vi "Format VI Info Table.vi"(5 "Type":T1=enum."LLB", 7 "Methods":T2, 8 "Error in":errorcluster caption="Error in (no error)", 9 "Msg Chain":string, 10 "VI Info Array":T3[](array[typedef]), 11 "VIDoc Printer - Confluence In":refnum<class "VIDoc Printer - Confluence.lvclass">) -> (0 "Error out":errorcluster, 2 "Table String":string, 3 "VIDoc Printer - Confluence Out":refnum<class "VIDoc Printer - Confluence.lvclass">)   [LabVIEW 2023, in "VIDoc Printer - Confluence.lvlib" / "VIDoc Printer - Confluence.lvclass"]
uses:
  VIDoc Printer - Confluence.lvclass
  Parsing/TypeDefs/Method Spec Cluster.ctl
  Parsing/TypeDefs/VI Type Extended Enum.ctl
  <vilib>/picture/picture.llb/imagedata.ctl
  Parsing/TypeDefs/Class Dispatch Type Enum.ctl
  Parsing/TypeDefs/Controls Info Cluster.ctl
  <vilib>/Utility/miscctls.llb/LVKeyTypeDef.ctl
  <vilib>/Utility/miscctls.llb/LVPointTypeDef.ctl
  Parsing/SubVIs/Structure Reporter/Tree Cluster.ctl
  Settings/Printer Settings/Detail Level Enum.ctl
  C:/projects/DMC/GitHub/DMC CLI VIDoc/Source/Documentation Generation/Printers/Printer/VIDoc Printer.lvclass
  Types/VI Method Types.ctl
  Printer/VIDoc Printer.lvclass/VIDoc Printer.ctl
  VIDoc Printer - Confluence.lvclass/VIDoc Printer - Confluence.ctl
  Types/VI Info Image Types.ctl
  Accessors/Get Method List Column Ordering - Minimal.vi
  Accessors/Get UI Column Ordering - Minimal.vi
  Accessors/Get VI Method Column Ordering - Minimal.vi
  Accessors/Get Class Method Column Ordering - Minimal.vi
  Accessors/Get Library Method Column Ordering - Minimal.vi
  Accessors/Get Interface Column Ordering - Minimal.vi
  Accessors/Get Method List Column Ordering - Standard.vi
  Accessors/Get UI Column Ordering - Standard.vi
  Accessors/Get VI Method Column Ordering - Standard.vi
  Accessors/Get Class Method Column Ordering - Standard.vi
  Accessors/Get Library Method Column Ordering - Standard.vi
  Accessors/Get Interface Column Ordering - Standard.vi
  Accessors/Get Method List Column Ordering - Full.vi
  Accessors/Get Library Method Column Ordering - Full.vi
  Accessors/Get UI Column Ordering - Full.vi
  Accessors/Get VI Method Column Ordering - Full.vi
  Accessors/Get Interface Column Ordering - Full.vi
  Accessors/Get Class Method Column Ordering - Full.vi
  Printer/Accessors/Get Formatting Settings.vi
  Accessors/Get Sortable Tables.vi
  Printer/VIDoc Printer.lvclass
  Confluence Formatting/Confluence Formatting.lvlib
  UI Interaction/UI Interaction.lvclass
  Parsing/VIDoc Parsing.lvlib
  Settings/Printer Settings/Printer Settings.lvclass
  Parsing/SubVIs/Structure Reporter/Structure Reporter.lvlib
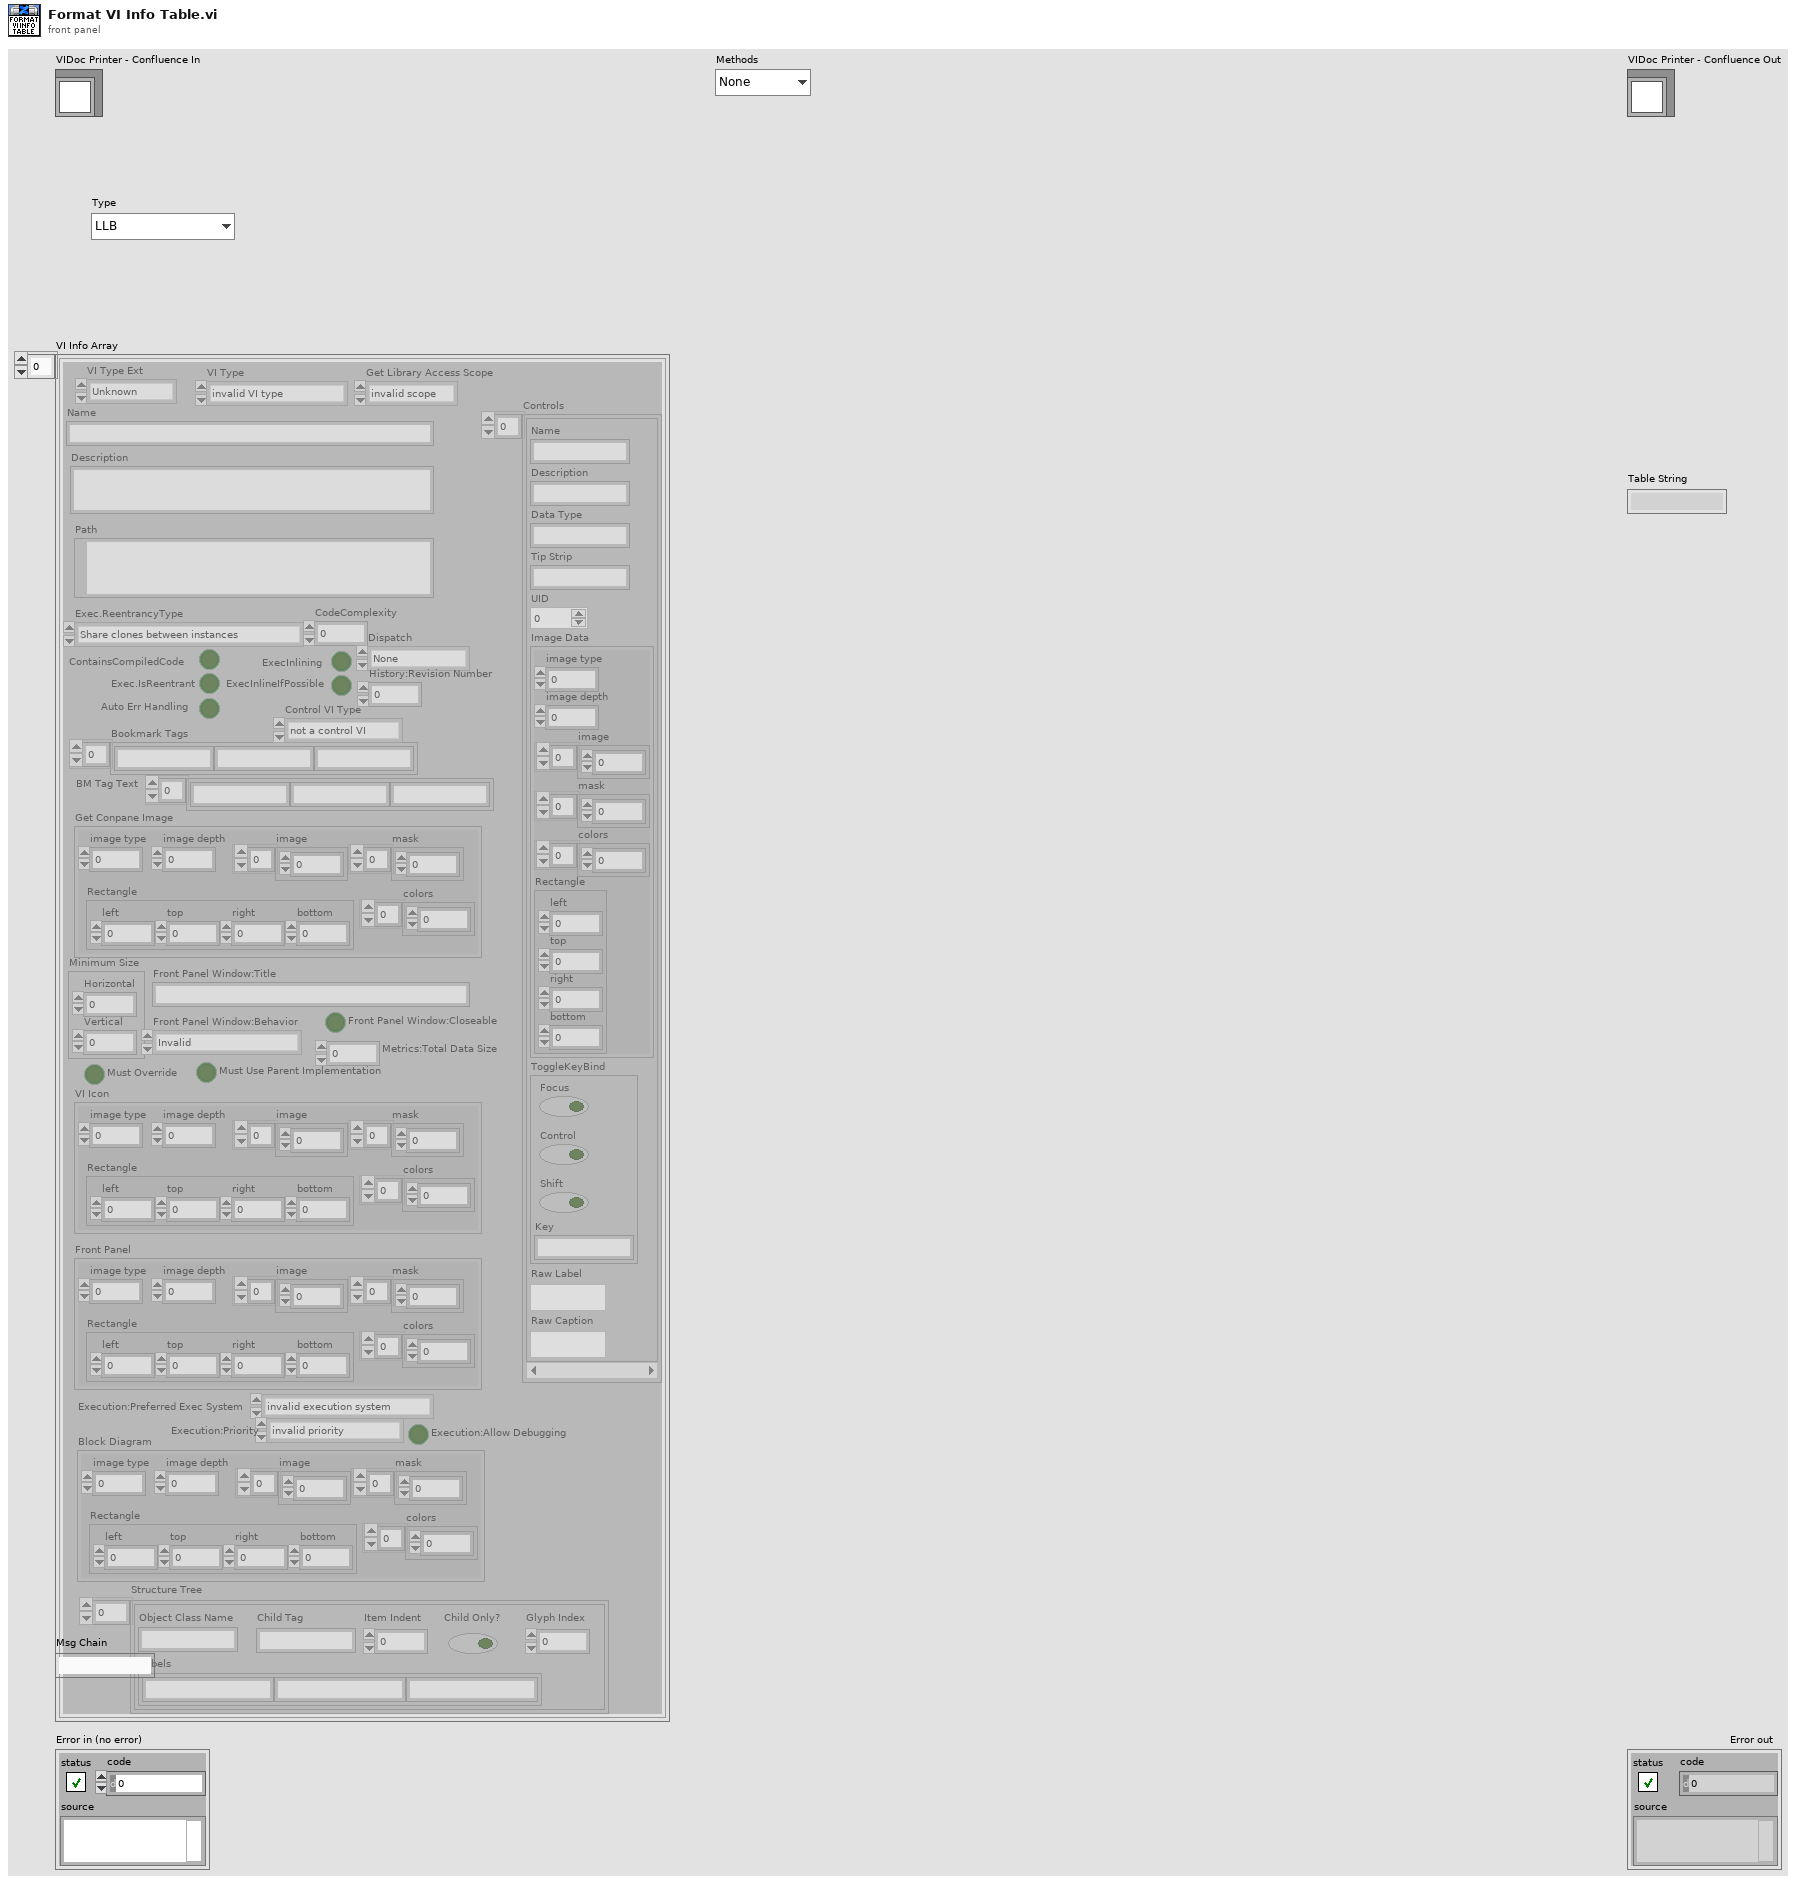
[diagram p1: front panel]
types:
  T1 = typedef "VIDoc Printer - Confluence.lvlib/VIDoc Printer - Confluence.lvclass/VI Method Types.ctl" = enum16{"Library", "Class", "Interface", "LLB", "UI", "List"}
  T2 = typedef "VIDoc Printer.lvlib/Printer Settings.lvclass/Detail Level Enum.ctl" = enum16{"None", "Minimal", "Standard", "Full"}
  T3 = typedef "VIDoc Parsing.lvlib/Method Spec Cluster.ctl" = cluster{"VI Type Ext":T4, "Name":string, "Path":path, "Get Conpane Image":T5, "Description":string, "Get Library Access Scope":enum32{"invalid scope", "public", "private", "protected", "community"}, "Dispatch":T6, "ContainsCompiledCode":bool, "Exec.IsReentrant":bool, "Exec.ReentrancyType":enum16{"Share clones between instances", "Preallocate clone for each instance"}, "ExecInlining":bool, "ExecInlineIfPossible":bool, "Auto Err Handling":bool, "CodeComplexity":sgl, "Bookmark Tags":string[], "Control VI Type":enum32{"not a control VI", "control", "typedef", "strict typedef"}, "Controls":T7[], "VI Type":enum32{"invalid VI type", "Standard VI", "Control VI", "Global VI", "Polymorphic VI", "Configuration VI", "SubSystem", "Facade VI", "Method VI", "Statechart Diagram VI"}, "Minimum Size":T9, "Front Panel Window:Title":string, "Front Panel Window:Behavior":enum32{"Invalid", "Default", "Floating", "Floating/Auto-Hide", "Modal"}, "Front Panel Window:Closeable":bool, "Must Override":bool, "Must Use Parent Implementation":bool, "VI Icon":T5, "Front Panel":T5, "History:Revision Number":u32, "Metrics:Total Data Size":u32, "Execution:Allow Debugging":bool, "Execution:Preferred Exec System":enum32{"invalid execution system", "user interface", "standard", "instrument i/o", "data acquisition", "other 1", "other 2", "same as caller"}, "Execution:Priority":enum32{"invalid priority", "background priority", "normal priority", "above normal priority", "high priority", "time critical priority", "subroutine"}, "BM Tag Text":string[], "Block Diagram":T5, "Structure Tree":T10[]}
  T4 = typedef "VIDoc Parsing.lvlib/VI Type Extended Enum.ctl" = enum16{"Unknown", "Class Method", "Class Accessor Get", "Class Accessor Set", "Class Control", "Library Method", "Library Control", "VI", "Control"}
  T5 = typedef "imagedata.ctl" = cluster{"image type":i32, "image depth":i32, "image":u8[], "mask":u8[], "colors":u32[], "Rectangle":cluster{"left":i16, "top":i16, "right":i16, "bottom":i16}}
  T6 = typedef "VIDoc Parsing.lvlib/Class Dispatch Type Enum.ctl" = enum16{"None", "Static", "Dynamic"}
  T7 = typedef "VIDoc Parsing.lvlib/Controls Info Cluster.ctl" = cluster{"Name":string, "Description":string, "Data Type":string, "Tip Strip":string, "UID":i32, "Image Data":T5, "ToggleKeyBind":T8, "Raw Label":string, "Raw Caption":string}
  T8 = typedef "LVKeyTypeDef.ctl" = cluster{"Focus":bool, "Control":bool, "Shift":bool, "Key":string}
  T9 = typedef "LVPointTypeDef.ctl" = cluster{"Horizontal":i16, "Vertical":i16}
  T10 = typedef "VIDoc Parsing.lvlib/Structure Reporter.lvlib/Tree Cluster.ctl" = cluster{"Object Class Name":string, "Labels":string[], "Child Tag":string, "Item Indent":i32, "Child Only?":bool, "Glyph Index":i32}
  T11 = typedef "VIDoc Printer - Confluence.lvlib/VIDoc Printer - Confluence.lvclass/VI Info Image Types.ctl" = enum16{"Conpane", "FP", "BD", "Icon"}
  T12 = typedef "VIDoc Printer.lvlib/Printer Settings.lvclass/Formatting Options.ctl" = cluster{"Background":cluster{"Public Scope":T13, "Protected Scope":T13, "Community Scope":T13, "Private Scope":T13, "Unknown Scope":T13, "Auto Error Handling":T13, "Inline":T13, "Separate CC":T13, "Execution Priority Normal":T13, "Reentrancy Non-RE":T13}, "Bookmark Options":T14}
  T13 = typedef "VIDoc Printer.lvlib/Printer Settings.lvclass/Background Formatting Cluster.ctl" = cluster{"Option":bool, "Color":u32, "Operator":bool}
  T14 = typedef "VIDoc Printer.lvlib/Printer Settings.lvclass/Bookmark Options.ctl" = cluster{"Bookmarks as New Line in VI Descriptions":bool, "Unique Bookmark Tags Only":bool, "Include Tag and Text":bool}
  T15 = typedef "VIDoc Printer - Confluence.lvlib/VIDoc Settings - Confluence.lvclass/VI Info Column.ctl" = enum16{"Name", "Conpane", "BD", "FP", "VI Icon", "Description", "Reentrant", "Inline", "Auto Error", "Compiled", "Code Complexity", "Data Size", "Debug", "Priority", "Rev", "Minimum Size", "Title", "FP Behavior", "FP Closeable", "Author", "Commit Hash", "Last Change", "Branch", "Scope", "Type", "Dispatch", "Must Override", "Must Use Parent", "Structure Tree"}
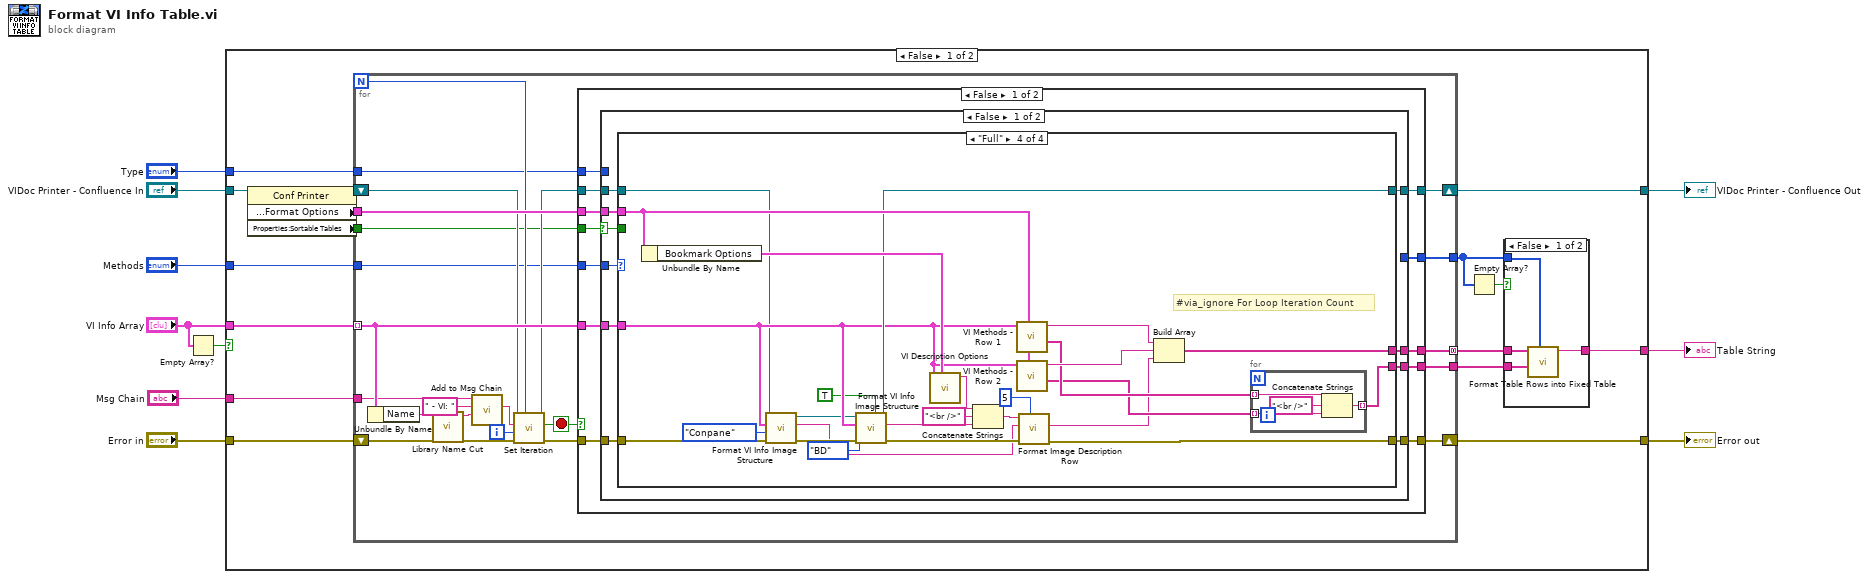
[diagram p0: block diagram]
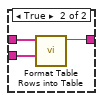
[diagram p2: hidden frame]
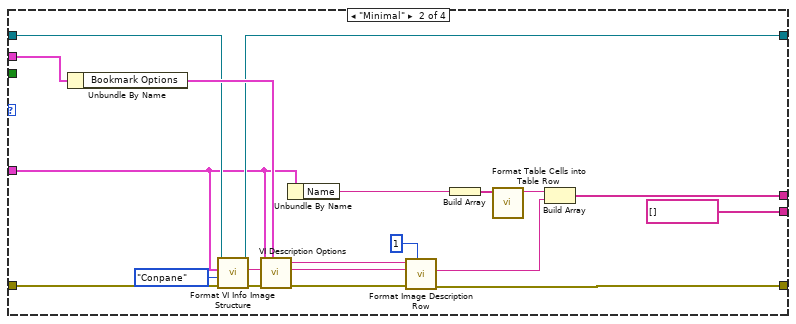
[diagram p4: hidden frame]
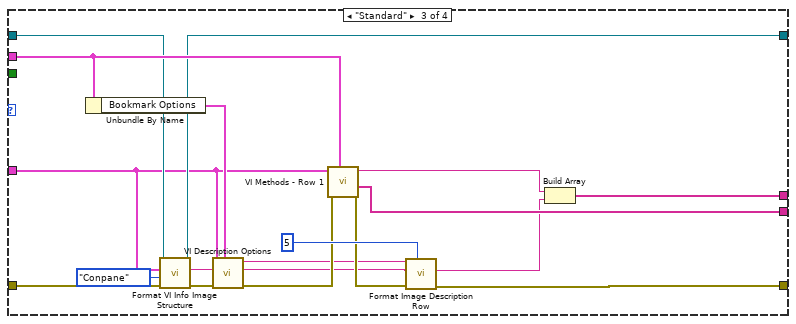
[diagram p5: hidden frame]
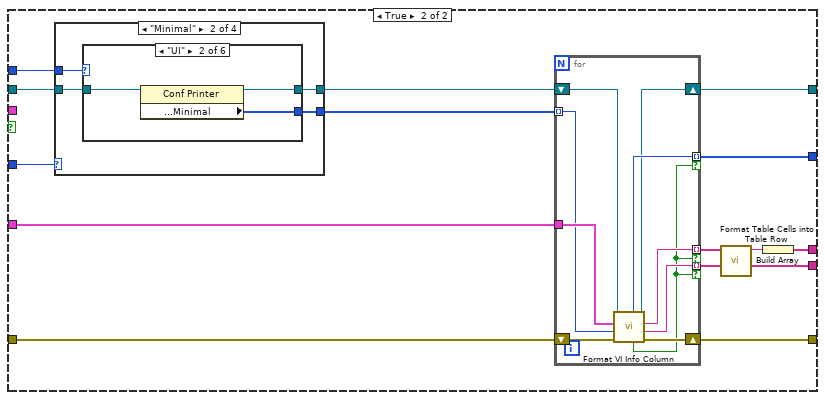
[diagram p6: hidden frame]
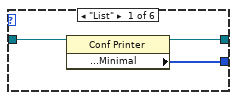
[diagram p8: hidden frame]
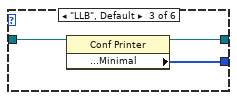
[diagram p9: hidden frame]
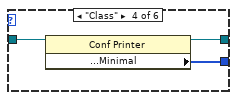
[diagram p10: hidden frame]
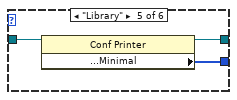
[diagram p11: hidden frame]
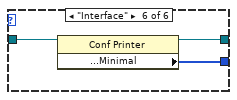
[diagram p12: hidden frame]
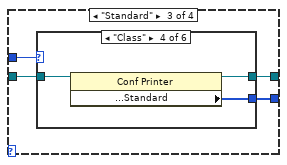
[diagram p13: hidden frame]
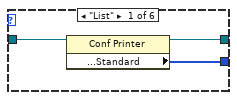
[diagram p14: hidden frame]
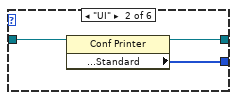
[diagram p15: hidden frame]
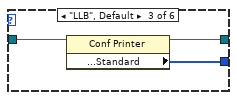
[diagram p16: hidden frame]
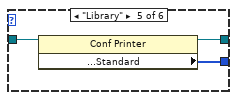
[diagram p17: hidden frame]
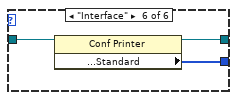
[diagram p18: hidden frame]
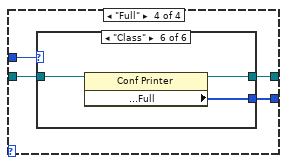
[diagram p19: hidden frame]
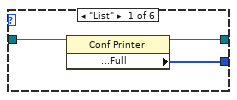
[diagram p20: hidden frame]
diagram:
  n1 = Empty Array?(array="VI Info Array") -> (empty?=w2:bool)
  n2 = case shown="False" w2 {
    tunnel: "Error in" -> [w25 w239]
    tunnel: [w24 w239] -> w9
    tunnel: [w23 _] -> w8
    tunnel: "VI Info Array" -> [w22 _]
    tunnel: "VIDoc Printer - Confluence In" -> [w21 w240]
    tunnel: [w20 w240] -> w6
    tunnel: "Msg Chain" -> [w19 _]
    tunnel: "Methods" -> [w18 _]
    tunnel: "Type" -> [w11 _]
    frame False {
      n3 = property class="Conf Printer"(reference=w21) -> (reference out=w16:refnum<class "VIDoc Printer - Confluence.lvclass">, "Properties:Settings:Formatting Options:Format Options"=w15:T12, "Properties:Sortable Tables"=w14:bool)  [unwired: 1 in, 1 out]
      n4 = for {
        N -> [w45]
        tunnel: w22 -> [w47] mode=indexing
        shift-right: [w54] -> w20
        shift-left: w16 -> [w43]
        shift-right: [w53] -> w24
        shift-left: w25 -> [w49]
        tunnel: w15 -> [w55]
        tunnel: [w52] -> w26 mode=concatenating
        tunnel: w19 -> [w46]
        tunnel: w18 -> [w40]
        tunnel: [w39] -> w17
        tunnel: w14 -> [w38]
        tunnel: [w37] -> w13
        tunnel: w11 -> [w36]
        i -> [w44]
        stop <- w41 stop-if-true
        n5 = Unbundle By Name(w47) -> ("Name"=w35:string)
        n6 = call "Library Name Cut.vi"("Name in"=w35) -> ("Name out"=w34:string)  [unwired: 10 in]
        n7 = call "Add to Msg Chain.vi"("New"=w34, "Separator (-)"=" - VI: ", "Msg Chain in"=w46) -> ("Msg Chain out"=w50:string)  [unwired: 8 in]
        n8 = call "Set Iteration.vi"("Progress Max"=w45, "error in (no error)"=w49, "Progress Value"=w44, "Message (No Message Update)"=w50, "VIDoc Printer In"=w43) -> ("error out"=w48:errorcluster, "Abort?"=w41:bool, "VIDoc Printer Out"=w42:refnum<class "VIDoc Printer - Confluence.lvclass">)  [unwired: 4 in]
        n9 = case shown="False" w41 {
          tunnel: w55 -> [w67 _]
          tunnel: [w66 w238] -> w54
          tunnel: [w65 w237] -> w53
          tunnel: [w64 _] -> w52
          tunnel: w48 -> [w63 w237]
          tunnel: w47 -> [w62 _]
          tunnel: w42 -> [w61 w238]
          tunnel: w40 -> [w60 _]
          tunnel: [w59 _] -> w39
          tunnel: w38 -> [w58 _]
          tunnel: [w57 _] -> w37
          tunnel: w36 -> [w56 _]
          frame False {
            n10 = case shown="False" w58 {
              selector: w58 -> [w68 _]
              tunnel: w67 -> [w77 _]
              tunnel: [w76 w152] -> w66
              tunnel: [w75 w158] -> w65
              tunnel: [w74 w154] -> w64
              tunnel: w63 -> [w73 w159]
              tunnel: w62 -> [w72 w151]
              tunnel: w61 -> [w71 w146]
              tunnel: w60 -> [w70 w150]
              tunnel: [w69 w157] -> w59
              tunnel: [_ w153] -> w57
              tunnel: w56 -> [_ w148]
              frame False {
                n11 = case shown="\"Full\"" w70 {
                  tunnel: w77 -> [_ w98 w113 w130]
                  tunnel: [w79 w85 w103 w126] -> w76
                  tunnel: [w78 w97 w116 w129] -> w75
                  tunnel: [_ w96 w115 w140] -> w74
                  tunnel: w73 -> [w78 w88 w106 w128]
                  tunnel: w72 -> [_ w81 w100 w123]
                  tunnel: w71 -> [w79 w84 w104 w117]
                  tunnel: [_ string[] [] w114 w135] -> w69
                  tunnel: w68 -> [_ _ _ _]
                  frame "None", Default {
                  }
                  frame "Minimal" {
                    n12 = Unbundle By Name(w98) -> ("Bookmark Options"=w89:T14)
                    n13 = call "Format VI Info Image Structure.vi"("Error in"=w88, "Image Type"=VI_Info_Image_Types."Conpane", "VI Info"=w81, "VIDoc Printer - Confluence In"=w84) -> ("Error out"=w86:errorcluster, "Image Structure Text"=w82:string, "VIDoc Printer - Confluence Out"=w85:refnum<class "VIDoc Printer - Confluence.lvclass">)  [unwired: 4 in, 1 out]
                    n14 = call "VI Description Options.vi"("Bookmark Options"=w89, "Error in"=w86, "VI Info"=w81) -> ("Error out"=w90:errorcluster, "Description"=w87:string)  [unwired: 7 in]
                    n15 = Unbundle By Name(w81) -> ("Name"=w83:string)
                    n16 = call "Format Image Description Row.vi"("Column Count"=1, "error in (no error)"=w90, "Image Structure"=w82, "Description"=w87) -> ("error out"=w97:errorcluster, "Table Row Text"=w91:string)  [unwired: 6 in]
                    n17 = Build Array(w83) -> (w94:string[])
                    n18 = call "Format Table Cells into Table Row.vi"("Table Cells"=w94) -> ("Table Row Text"=w92:string)  [unwired: 10 in]
                    n19 = Build Array(w92, w91) -> (w96:string[])
                  }
                  frame "Standard" {
                    n20 = Unbundle By Name(w113) -> ("Bookmark Options"=w107:T14)
                    n21 = call "Format VI Info Image Structure.vi"("Error in"=w106, "Image Type"=VI_Info_Image_Types."Conpane", "VI Info"=w100, "VIDoc Printer - Confluence In"=w104) -> ("Error out"=w105:errorcluster, "Image Structure Text"=w101:string, "VIDoc Printer - Confluence Out"=w103:refnum<class "VIDoc Printer - Confluence.lvclass">)  [unwired: 4 in, 1 out]
                    n22 = call "VI Description Options.vi"("Bookmark Options"=w107, "Error in"=w105, "VI Info"=w100) -> ("Error out"=w110:errorcluster, "Description"=w102:string)  [unwired: 7 in]
                    n23 = call "VI Methods - Row 1.vi"("Format Options"=w113, "Error in"=w110, "VI Info"=w100) -> ("Error out"=w109:errorcluster, "Column Headers"=w114:string[], "Table Row Text"=w108:string)  [unwired: 6 in]
                    n24 = call "Format Image Description Row.vi"("Column Count"=5, "error in (no error)"=w109, "Image Structure"=w101, "Description"=w102) -> ("error out"=w116:errorcluster, "Table Row Text"=w111:string)  [unwired: 6 in]
                    n25 = Build Array(w108, w111) -> (w115:string[])
                  }
                  frame "Full" {
                    # "#via_ignore For Loop Iteration Count"
                    n26 = Unbundle By Name(w130) -> ("Bookmark Options"=w131:T14)
                    n27 = call "Format VI Info Image Structure.vi"("Error in"=w128, "Image Type"=VI_Info_Image_Types."Conpane", "VI Info"=w123, "VIDoc Printer - Confluence In"=w117) -> ("Image Structure Text"=w119:string, "VIDoc Printer - Confluence Out"=w118:refnum<class "VIDoc Printer - Confluence.lvclass">)  [unwired: 4 in, 2 out]
                    n28 = call "Format VI Info Image Structure.vi"("Wrap with Expand? (F)"=TRUE, "Error in"=w128, "Image Type"=VI_Info_Image_Types."BD", "VI Info"=w123, "VIDoc Printer - Confluence In"=w118) -> ("Error out"=w127:errorcluster, "Image Structure Text"=w120:string, "VIDoc Printer - Confluence Out"=w126:refnum<class "VIDoc Printer - Confluence.lvclass">)  [unwired: 3 in, 1 out]
                    n29 = call "VI Description Options.vi"("Bookmark Options"=w131, "VI Info"=w123) -> ("Description"=w133:string)  [unwired: 8 in, 1 out]
                    n30 = Concatenate Strings(w133, "<br />" ("string"), w120) -> (w125:string)
                    n31 = call "VI Methods - Row 1.vi"("Format Options"=w130, "VI Info"=w123) -> ("Column Headers"=w137:string[], "Table Row Text"=w139:string)  [unwired: 7 in, 1 out]
                    n32 = call "VI Methods - Row 2.vi"("Format Options"=w130, "VI Info"=w123) -> ("Column Headers"=w136:string[], "Table Row Text"=w138:string)  [unwired: 7 in, 1 out]
                    n33 = call "Format Image Description Row.vi"("Column Count"=5, "error in (no error)"=w127, "Image Structure"=w119, "Description"=w125) -> ("error out"=w129:errorcluster, "Table Row Text"=w132:string)  [unwired: 6 in]
                    n34 = Build Array(w139, w138, w132) -> (w140:string[])
                    n35 = for {
                      tunnel: w137 -> [w145] mode=indexing
                      tunnel: w136 -> [w144] mode=indexing
                      tunnel: [w143] -> w135 mode=indexing
                      n36 = Concatenate Strings(w145, "<br />" ("string"), w144) -> (w143:string)
                    }
                  }
                }
              }
              frame True {
                n37 = case shown="\"Minimal\"" w150 {
                  tunnel: [_ w164 w186 w208] -> w149
                  tunnel: w148 -> [_ w163 w185 w207]
                  tunnel: [w160 w162 w184 w206] -> w147
                  tunnel: w146 -> [w160 w161 w183 w205]
                  frame "None", Default {
                  }
                  frame "Minimal" {
                    n38 = case shown="\"UI\"" w163 {
                      tunnel: [w165 w168 w171 w174 w177 w180] -> w164
                      tunnel: [w166 w169 w172 w175 w178 w181] -> w162
                      tunnel: w161 -> [w167 w170 w173 w176 w179 w182]
                      frame "List" {
                        n39 = property class="Conf Printer"(reference=w167) -> (reference out=w166:refnum<class "VIDoc Printer - Confluence.lvclass">, "Properties:Table Column Ordering:Method List:Minimal"=w165:T15[])  [unwired: 1 in, 1 out]
                      }
                      frame "UI" {
                        n40 = property class="Conf Printer"(reference=w170) -> (reference out=w169:refnum<class "VIDoc Printer - Confluence.lvclass">, "Properties:Table Column Ordering:UI:Minimal"=w168:T15[])  [unwired: 1 in, 1 out]
                      }
                      frame "LLB", Default {
                        n41 = property class="Conf Printer"(reference=w173) -> (reference out=w172:refnum<class "VIDoc Printer - Confluence.lvclass">, "Properties:Table Column Ordering:VI Method:Minimal"=w171:T15[])  [unwired: 1 in, 1 out]
                      }
                      frame "Class" {
                        n42 = property class="Conf Printer"(reference=w176) -> (reference out=w175:refnum<class "VIDoc Printer - Confluence.lvclass">, "Properties:Table Column Ordering:Class Method:Minimal"=w174:T15[])  [unwired: 1 in, 1 out]
                      }
                      frame "Library" {
                        n43 = property class="Conf Printer"(reference=w179) -> (reference out=w178:refnum<class "VIDoc Printer - Confluence.lvclass">, "Properties:Table Column Ordering:Library Method:Minimal"=w177:T15[])  [unwired: 1 in, 1 out]
                      }
                      frame "Interface" {
                        n44 = property class="Conf Printer"(reference=w182) -> (reference out=w181:refnum<class "VIDoc Printer - Confluence.lvclass">, "Properties:Table Column Ordering:Interface:Minimal"=w180:T15[])  [unwired: 1 in, 1 out]
                      }
                    }
                  }
                  frame "Standard" {
                    n45 = case shown="\"Class\"" w185 {
                      tunnel: [w187 w190 w193 w196 w199 w202] -> w186
                      tunnel: [w188 w191 w194 w197 w200 w203] -> w184
                      tunnel: w183 -> [w189 w192 w195 w198 w201 w204]
                      frame "List" {
                        n46 = property class="Conf Printer"(reference=w189) -> (reference out=w188:refnum<class "VIDoc Printer - Confluence.lvclass">, "Properties:Table Column Ordering:Method List:Standard"=w187:T15[])  [unwired: 1 in, 1 out]
                      }
                      frame "UI" {
                        n47 = property class="Conf Printer"(reference=w192) -> (reference out=w191:refnum<class "VIDoc Printer - Confluence.lvclass">, "Properties:Table Column Ordering:UI:Standard"=w190:T15[])  [unwired: 1 in, 1 out]
                      }
                      frame "LLB", Default {
                        n48 = property class="Conf Printer"(reference=w195) -> (reference out=w194:refnum<class "VIDoc Printer - Confluence.lvclass">, "Properties:Table Column Ordering:VI Method:Standard"=w193:T15[])  [unwired: 1 in, 1 out]
                      }
                      frame "Class" {
                        n49 = property class="Conf Printer"(reference=w198) -> (reference out=w197:refnum<class "VIDoc Printer - Confluence.lvclass">, "Properties:Table Column Ordering:Class Method:Standard"=w196:T15[])  [unwired: 1 in, 1 out]
                      }
                      frame "Library" {
                        n50 = property class="Conf Printer"(reference=w201) -> (reference out=w200:refnum<class "VIDoc Printer - Confluence.lvclass">, "Properties:Table Column Ordering:Library Method:Standard"=w199:T15[])  [unwired: 1 in, 1 out]
                      }
                      frame "Interface" {
                        n51 = property class="Conf Printer"(reference=w204) -> (reference out=w203:refnum<class "VIDoc Printer - Confluence.lvclass">, "Properties:Table Column Ordering:Interface:Standard"=w202:T15[])  [unwired: 1 in, 1 out]
                      }
                    }
                  }
                  frame "Full" {
                    n52 = case shown="\"Class\"" w207 {
                      tunnel: [w209 w212 w215 w218 w221 w224] -> w208
                      tunnel: [w210 w213 w216 w219 w222 w225] -> w206
                      tunnel: w205 -> [w211 w214 w217 w220 w223 w226]
                      frame "List" {
                        n53 = property class="Conf Printer"(reference=w211) -> (reference out=w210:refnum<class "VIDoc Printer - Confluence.lvclass">, "Properties:Table Column Ordering:Method List:Full"=w209:T15[])  [unwired: 1 in, 1 out]
                      }
                      frame "Library" {
                        n54 = property class="Conf Printer"(reference=w214) -> (reference out=w213:refnum<class "VIDoc Printer - Confluence.lvclass">, "Properties:Table Column Ordering:Library Method:Full"=w212:T15[])  [unwired: 1 in, 1 out]
                      }
                      frame "UI" {
                        n55 = property class="Conf Printer"(reference=w217) -> (reference out=w216:refnum<class "VIDoc Printer - Confluence.lvclass">, "Properties:Table Column Ordering:UI:Full"=w215:T15[])  [unwired: 1 in, 1 out]
                      }
                      frame "LLB" {
                        n56 = property class="Conf Printer"(reference=w220) -> (reference out=w219:refnum<class "VIDoc Printer - Confluence.lvclass">, "Properties:Table Column Ordering:VI Method:Full"=w218:T15[])  [unwired: 1 in, 1 out]
                      }
                      frame "Interface" {
                        n57 = property class="Conf Printer"(reference=w223) -> (reference out=w222:refnum<class "VIDoc Printer - Confluence.lvclass">, "Properties:Table Column Ordering:Interface:Full"=w221:T15[])  [unwired: 1 in, 1 out]
                      }
                      frame "Class" {
                        n58 = property class="Conf Printer"(reference=w226) -> (reference out=w225:refnum<class "VIDoc Printer - Confluence.lvclass">, "Properties:Table Column Ordering:Class Method:Full"=w224:T15[])  [unwired: 1 in, 1 out]
                      }
                    }
                  }
                }
                n59 = for {
                  shift-right: [w235] -> w158
                  shift-left: w159 -> [w236]
                  tunnel: [w234] -> w157 mode=indexing if=w227
                  tunnel: [w233] -> w156 mode=indexing if=w227
                  tunnel: [w232] -> w153 mode=indexing if=w227
                  shift-right: [w230] -> w152
                  shift-left: w147 -> [w231]
                  tunnel: w151 -> [w229]
                  tunnel: w149 -> [w228] mode=indexing
                  n60 = call "Format VI Info Column.vi"("error in (no error)"=w236, "Column"=w228, "VI Info"=w229, "VIDoc Printer - Confluence In"=w231) -> ("error out"=w235:errorcluster, "Header"=w234:string, "Cell Text"=w233:string, "VIDoc Printer - Confluence Out"=w230:refnum<class "VIDoc Printer - Confluence.lvclass">, "Viable Value?"=w227:bool, "Pixel Width"=w232:i16)  [unwired: 2 in]
                }
                n61 = call "Format Table Cells into Table Row.vi"("Table Cells"=w156) -> ("Table Row Text"=w155:string)  [unwired: 10 in]
                n62 = Build Array(w155) -> (w154:string[])
              }
            }
          }
          frame True {
          }
        }
      }
      n63 = Empty Array?(array=w13) -> (empty?=w12:bool)
      n64 = case shown="False" w12 {
        tunnel: w26 -> [w29 w33]
        tunnel: [w27 w32] -> w23
        tunnel: w17 -> [w30 w31]
        tunnel: w13 -> [w28 _]
        frame False {
          n65 = call "Format Table Rows into Fixed Table.vi"("Column Pixel Widths"=w28, "Table Headers"=w30, "Table Rows"=w29) -> ("Table Text"=w27:string)  [unwired: 8 in]
        }
        frame True {
          n66 = call "Format Table Rows into Table.vi"("Table Headers"=w31, "Table Rows"=w33) -> ("Table Text"=w32:string)  [unwired: 9 in]
        }
      }
    }
    frame True {
    }
  }
  "Error out" <- w9
  "Table String" <- w8
  "VIDoc Printer - Confluence Out" <- w6
